vi "AlGaInPAs_prep_run_cont_v09.vi"(2 "Debug Mode":bool, 3 "Elapsed Time(s)":dbl, 4 "State":enum16{"Edit", "Start", "Run", "End", "Idle"}(ring), 5 "Argument List In":string[](array[string])) -> (0 "Status Out":string, 1 "Argument List Out":string[](array[string]))   [LabVIEW 2011]
panel:
  out "Prep-In var":bool
  out "Prep-Ga var":bool
  out "Prep-Al var":bool
  out "Prep-P var":bool
  out "Prep-As var":bool
  out "prep_done":bool
  out "run started":bool
  out "first":bool=TRUE
  out "total time":dbl
  out "is OK?":bool
  out "AsH3?":bool
  out "PH3?":bool
  out "In?":bool
  out "Ga?":bool
  out "Al?":bool
  in  "Prep As":bool caption="Pre-run"
  in  "Prep P":bool caption="Pre-run"
  in  "Prep In":bool caption="Pre-run"
  in  "Prep Ga":bool caption="Pre-run"
  in  "prep_time":dbl caption="pre-run time (s)"
  in  "Prep Al":bool caption="Pre-run"
  in  "Run As":bool caption="Run"
  in  "AsH3 Flow":dbl caption="AsH3 Flow (0-10 sccm)" format="%.2f"
  in  "P Flow":dbl caption="P Flow (0-100 sccm)" format="%.2f"
  in  "Run P":bool caption="Run"
  in  "In Flow":dbl caption="In Flow (0-100 sscm)" format="%.2f"
  in  "Run In":bool caption="Run"
  in  "Run Ga":bool caption="Run"
  in  "Ga Flow":dbl caption="Ga Flow (0-10 sscm)" format="%.2f"
  in  "Run Al":bool caption="Run"
  in  "Al Flow":dbl caption="Al Flow (0-100 sscm)" format="%.2f"
  in  "Cancel":bool
  in  "OK":bool
  out "tTotal(s) 2":dbl
  # "Add pre-run time to run time in editor."
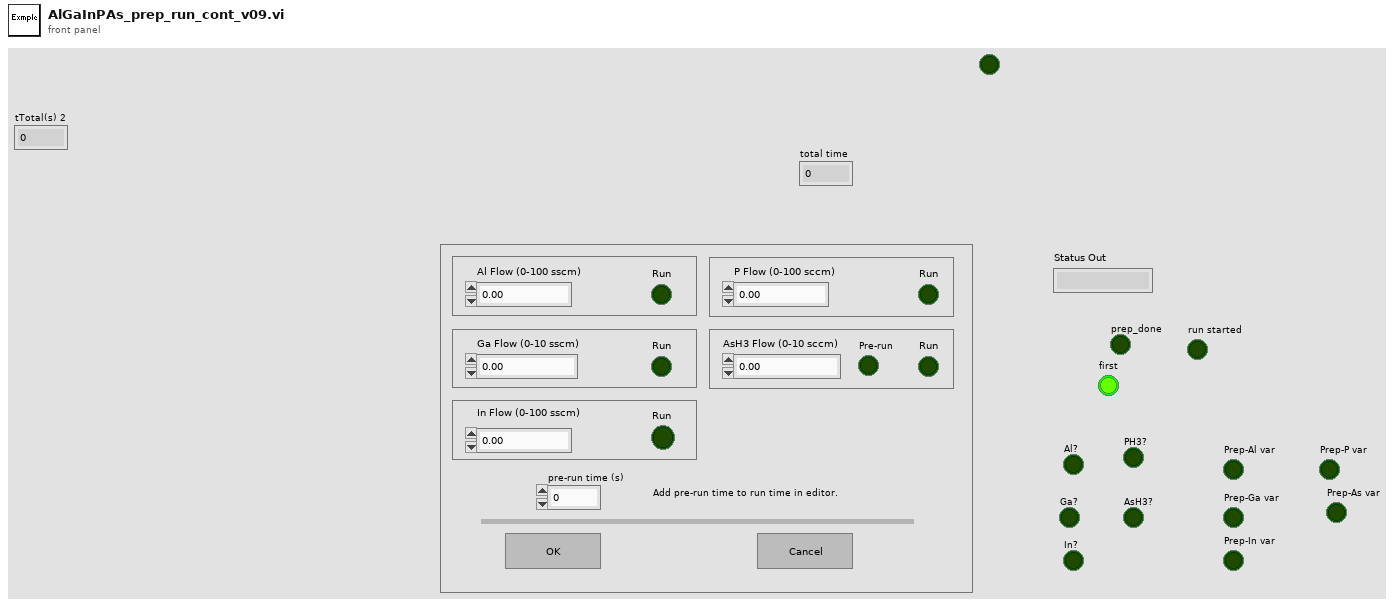
[diagram p1: front panel]
types:
  T1 = enum16{"Discrete", "Continuous", "Instantaneous", "Finite"}
  T2 = enum32{"Invalid", "Default", "Floating", "Floating/Auto-Hide", "Modal"}
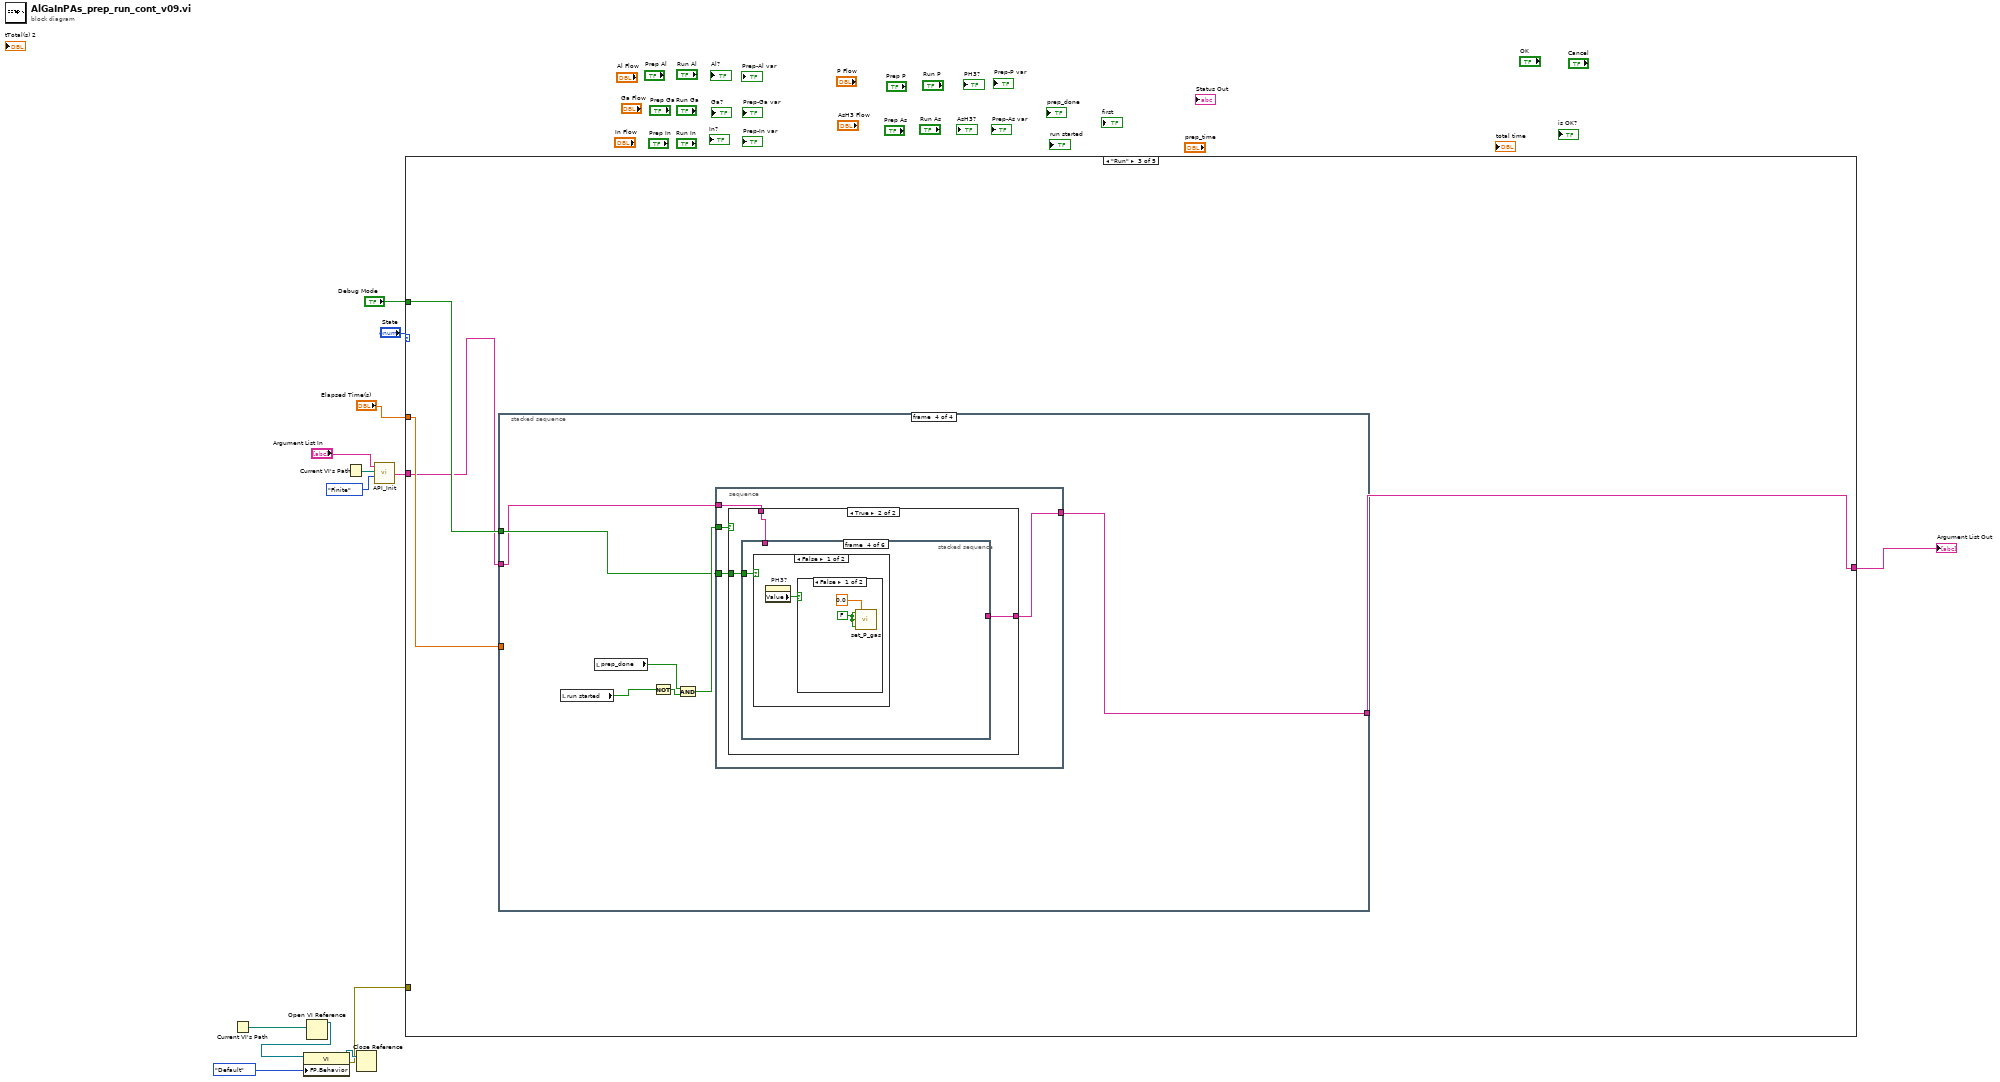
[diagram p0: block diagram]
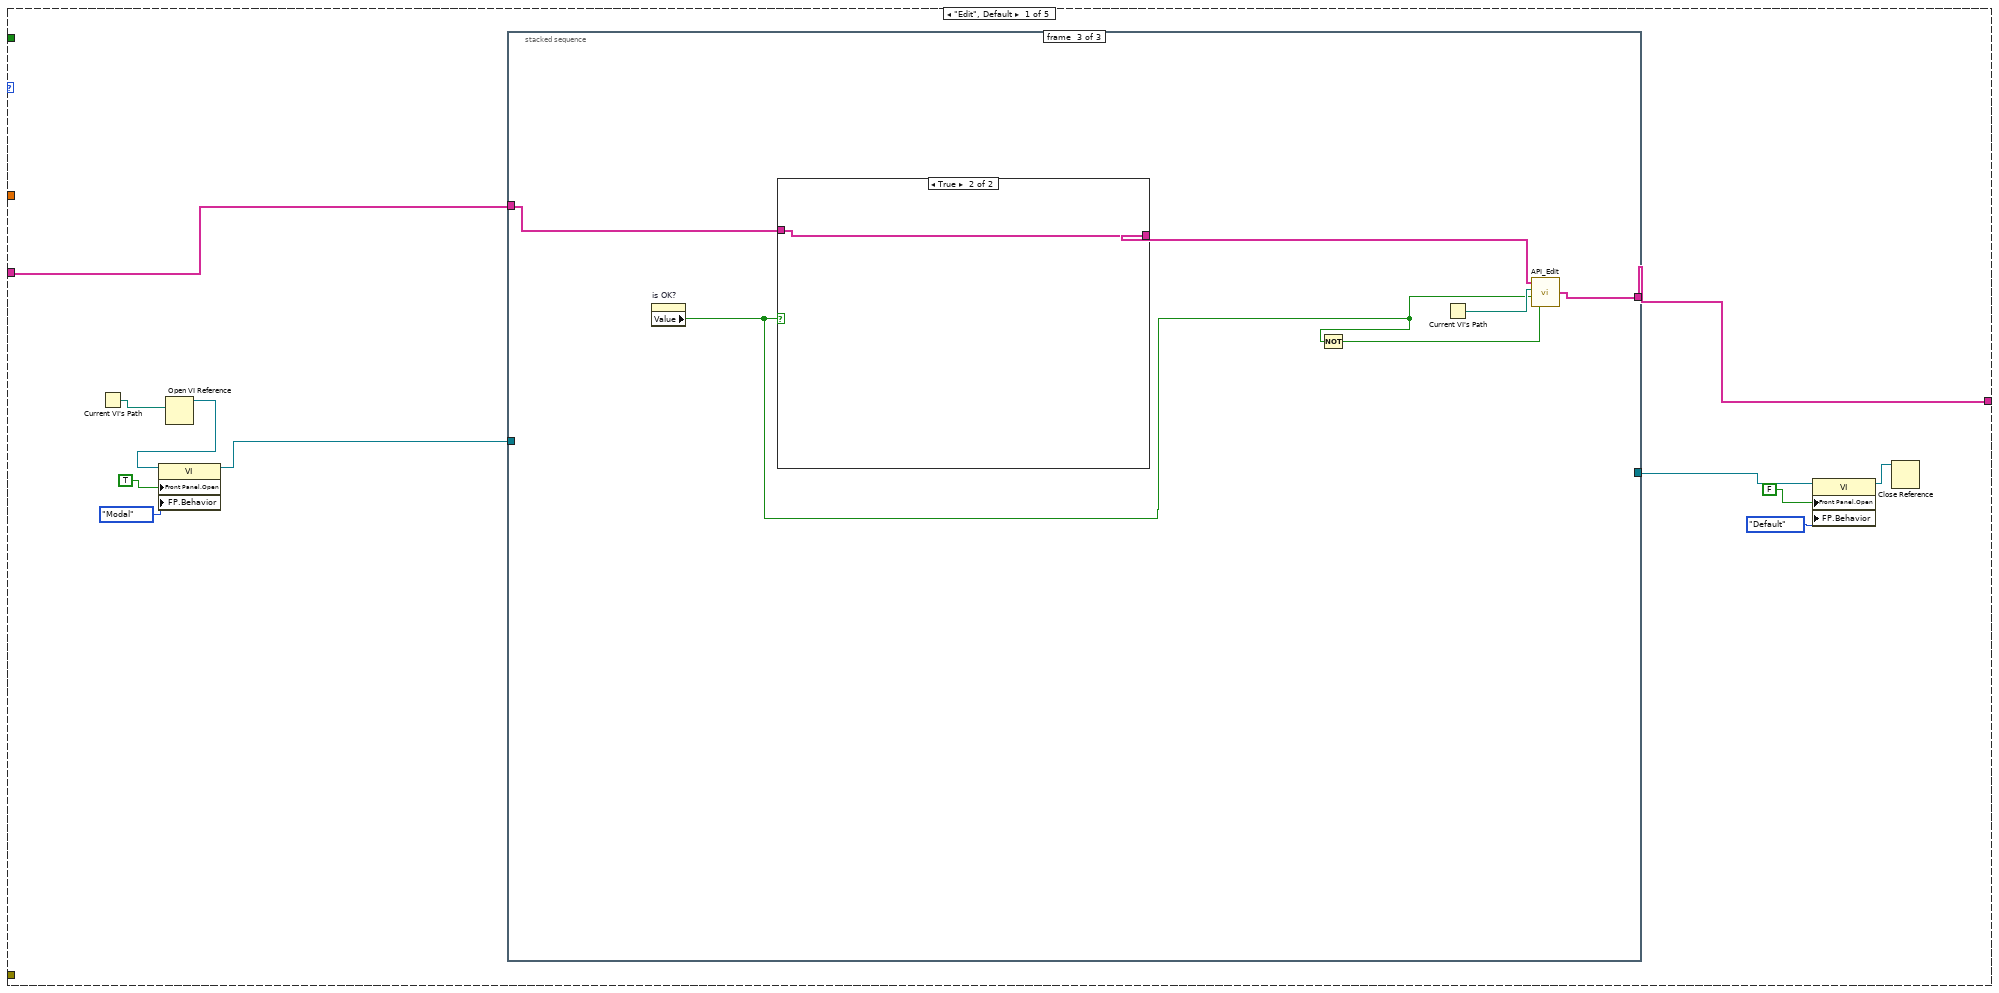
[diagram p2: hidden frame]
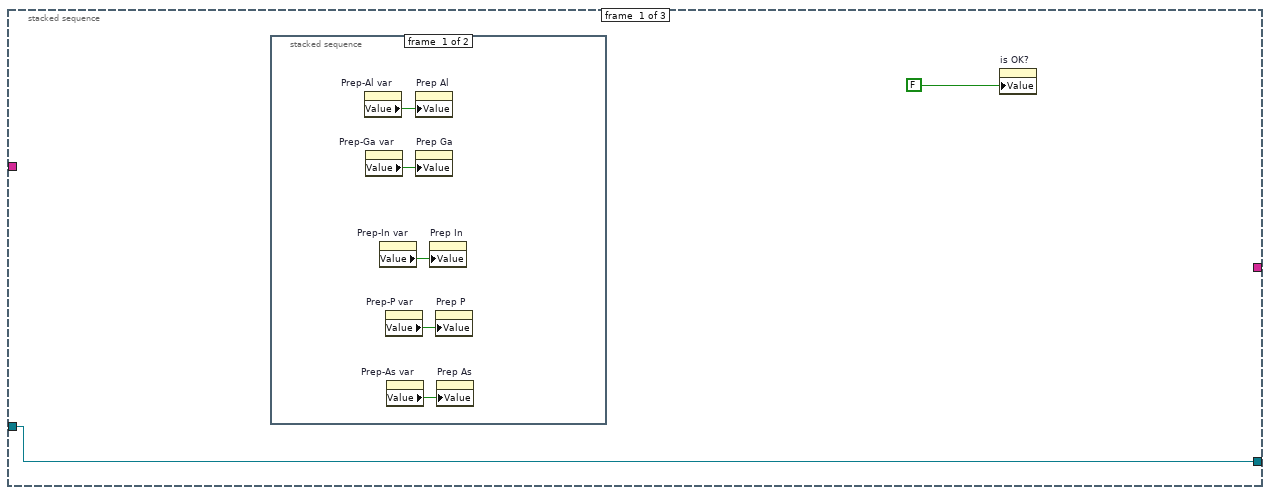
[diagram p3: hidden frame]
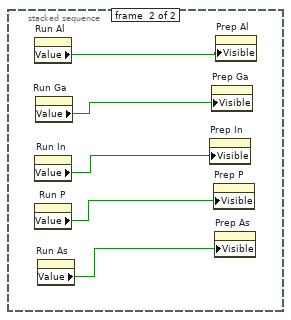
[diagram p4: hidden frame]
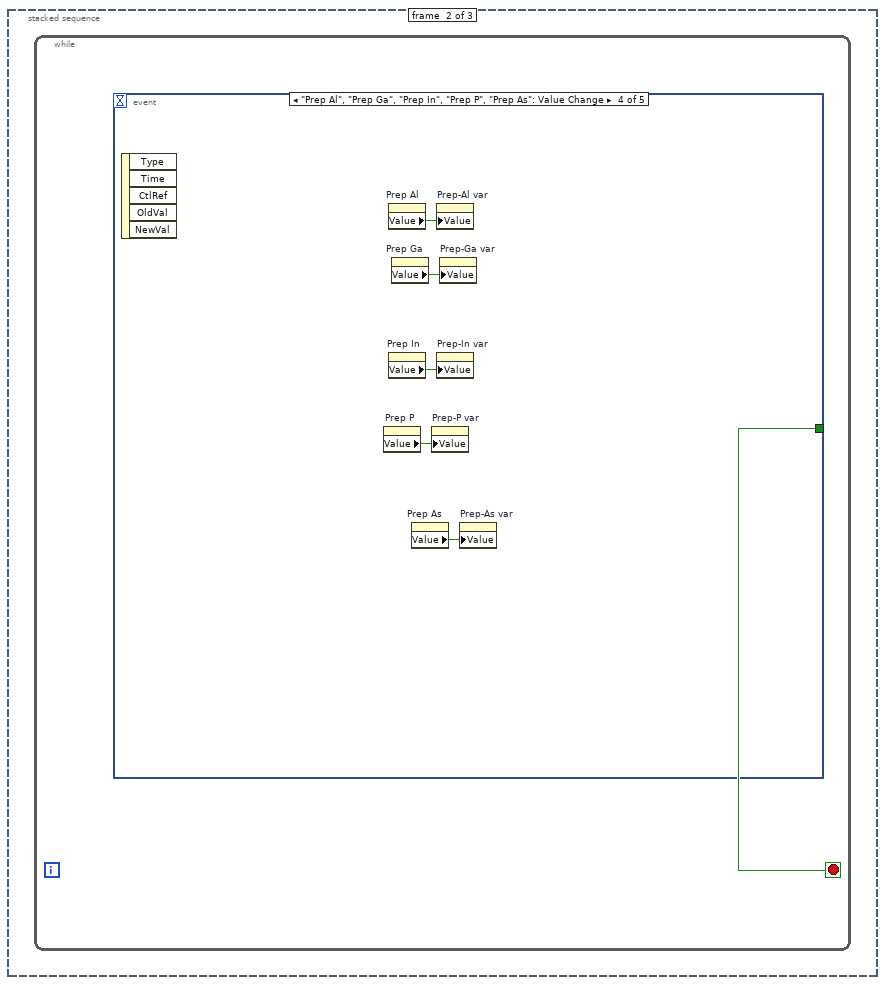
[diagram p5: hidden frame]
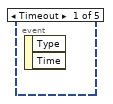
[diagram p6: hidden frame]
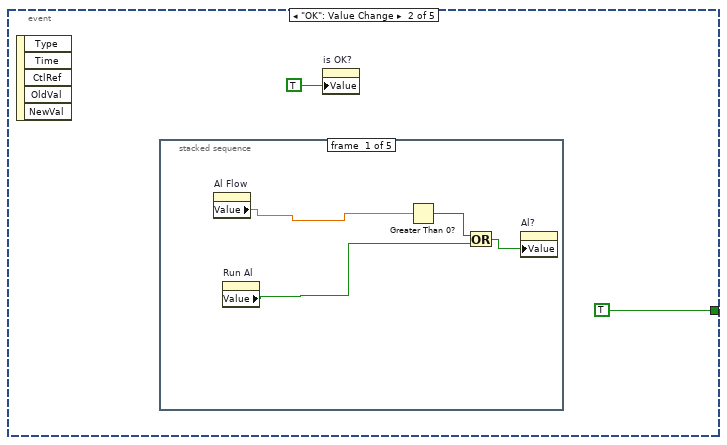
[diagram p7: hidden frame]
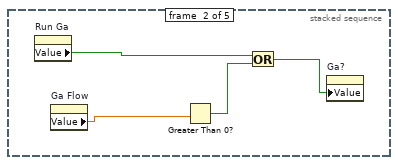
[diagram p8: hidden frame]
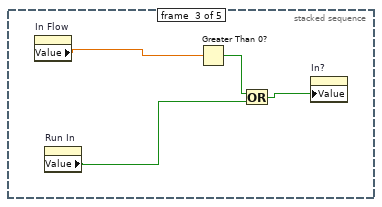
[diagram p9: hidden frame]
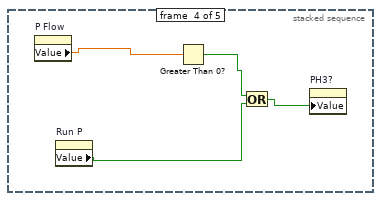
[diagram p10: hidden frame]
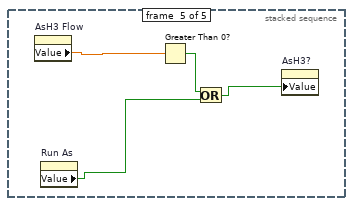
[diagram p11: hidden frame]
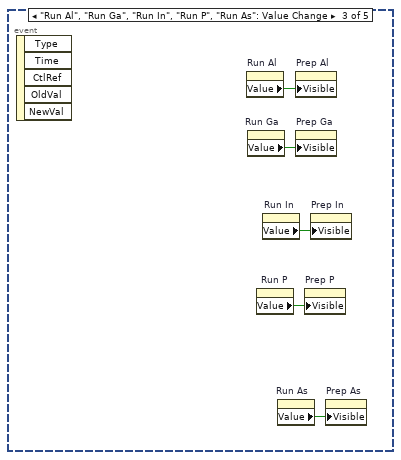
[diagram p12: hidden frame]
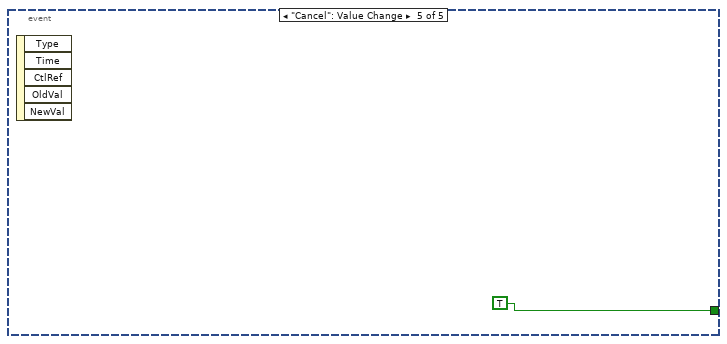
[diagram p13: hidden frame]
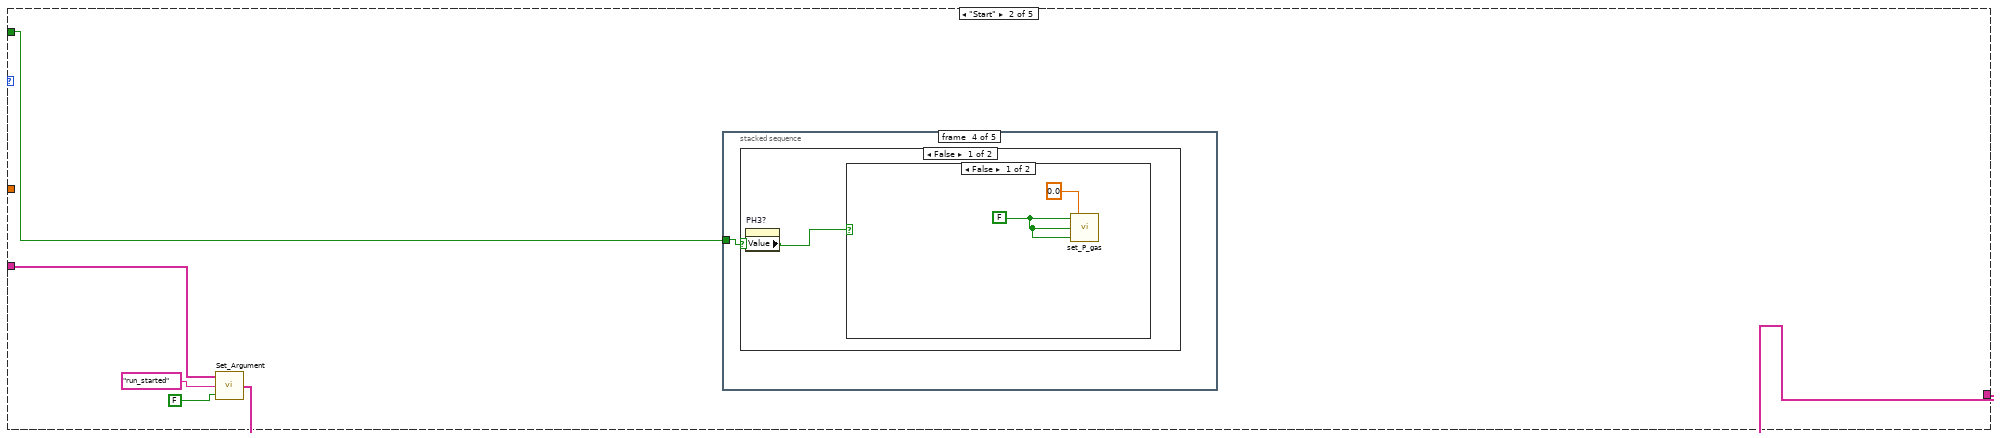
[diagram p15: hidden frame]
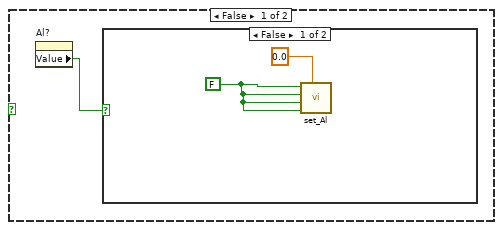
[diagram p17: hidden frame]
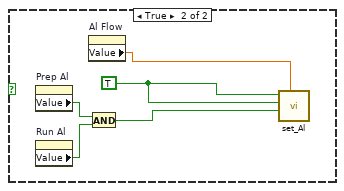
[diagram p18: hidden frame]
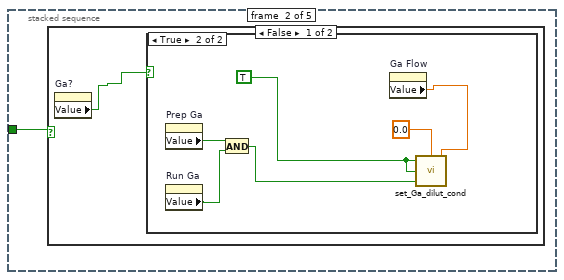
[diagram p19: hidden frame]
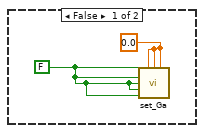
[diagram p20: hidden frame]
diagram:
  n1 = Current VI's Path() -> (path=w9:path)
  n2 = Open VI Reference(vi path=w9) -> (vi reference=w8:refnum<vi>)  [unwired: 1 in, 5 out]
  n3 = property class="VI"(reference=w8, "FP.Behavior"=T2."Default" ("Front Panel Window:Behavior")) -> (reference out=w6:refnum<vi>, error out=w5:errorcluster)  [unwired: 1 in]
  n4 = Current VI's Path() -> (path=w4:path)
  n5 = Close Reference(reference=w6) -> ()  [unwired: 1 in, 1 out]
  n6 = call "API_Init.vi"("API Mode"=T1."Finite", "VI Path"=w4, "Argument List In"="Argument List In") -> ("Argument List Out"=w1:string[])  [unwired: 1 in]
  n7 = case shown="\"Run\"" "State" {
    tunnel: "Debug Mode" -> [_ w79 w131 _ _]
    tunnel: "Elapsed Time(s)" -> [_ _ w133 _ _]
    tunnel: w1 -> [w15 w81 w130 w246 w247]
    tunnel: [w14 w80 w132 w246 w247] -> w10
    tunnel: w5 -> [_ _ _ _ _]
    frame "Edit", Default {
      n8 = Current VI's Path() -> (path=w20:path)
      n9 = Open VI Reference(vi path=w20) -> (vi reference=w19:refnum<vi>)  [unwired: 1 in, 5 out]
      n10 = property class="VI"(reference=w19, "Front Panel.Open"=TRUE ("Front Panel Window:Open"), "FP.Behavior"=T2."Modal" ("Front Panel Window:Behavior")) -> (reference out=w18:refnum<vi>)  [unwired: 1 in, 1 out]
      n11 = stacked-sequence {
        tunnel: w15 -> [_ _ w74]
        tunnel: w18 -> [w26 _ _]
        tunnel: [w26 _ _] -> w22
        tunnel: [_ _ w72] -> w14
        frame #0 {
          n12 = stacked-sequence {
            frame #0 {
              n13 = property on="Prep-Al var" class="Bool (strict)"() -> ("Value"=w31:bool)  [unwired: 2 in, 2 out]
              n14 = property on="Prep-Ga var" class="Bool (strict)"() -> ("Value"=w30:bool)  [unwired: 2 in, 2 out]
              n15 = property on="Prep-In var" class="Bool (strict)"() -> ("Value"=w29:bool)  [unwired: 2 in, 2 out]
              n16 = property on="Prep-P var" class="Bool (strict)"() -> ("Value"=w28:bool)  [unwired: 2 in, 2 out]
              n17 = property on="Prep-As var" class="Bool (strict)"() -> ("Value"=w27:bool)  [unwired: 2 in, 2 out]
              n18 = property on="Prep Al" class="Bool (strict)"("Value"=w31) -> ()  [unwired: 2 in, 2 out]
              n19 = property on="Prep Ga" class="Bool (strict)"("Value"=w30) -> ()  [unwired: 2 in, 2 out]
              n20 = property on="Prep In" class="Bool (strict)"("Value"=w29) -> ()  [unwired: 2 in, 2 out]
              n21 = property on="Prep P" class="Bool (strict)"("Value"=w28) -> ()  [unwired: 2 in, 2 out]
              n22 = property on="Prep As" class="Bool (strict)"("Value"=w27) -> ()  [unwired: 2 in, 2 out]
            }
            frame #1 {
              n23 = property on="Run Al" class="Bool (strict)"() -> ("Value"=w36:bool)  [unwired: 2 in, 2 out]
              n24 = property on="Run In" class="Bool (strict)"() -> ("Value"=w34:bool)  [unwired: 2 in, 2 out]
              n25 = property on="Run P" class="Bool (strict)"() -> ("Value"=w33:bool)  [unwired: 2 in, 2 out]
              n26 = property on="Run Ga" class="Bool (strict)"() -> ("Value"=w35:bool)  [unwired: 2 in, 2 out]
              n27 = property on="Run As" class="Bool (strict)"() -> ("Value"=w32:bool)  [unwired: 2 in, 2 out]
              n28 = property on="Prep In" class="Bool (strict)"("Visible"=w34) -> ()  [unwired: 2 in, 2 out]
              n29 = property on="Prep Ga" class="Bool (strict)"("Visible"=w35) -> ()  [unwired: 2 in, 2 out]
              n30 = property on="Prep P" class="Bool (strict)"("Visible"=w33) -> ()  [unwired: 2 in, 2 out]
              n31 = property on="Prep As" class="Bool (strict)"("Visible"=w32) -> ()  [unwired: 2 in, 2 out]
              n32 = property on="Prep Al" class="Bool (strict)"("Visible"=w36) -> ()  [unwired: 2 in, 2 out]
            }
          }
          n33 = property on="is OK?" class="Bool (strict)"("Value"=FALSE ("is OK?")) -> ()  [unwired: 2 in, 2 out]
        }
        frame #1 {
          n34 = while {
            stop <- w37 stop-if-true
            n35 = event shown="[3] \"Prep Al\", \"Prep Ga\", \"Prep In\", \"Prep P\", \"Prep As\": Value Change" {
              selector: _ -> [_ _ _ _ _]
              dyn-events: _ -> [_ _ _ _ _]
              timeout: _ -> [_ _ _ _ _]
              tunnel: [_ TRUE _ _ TRUE] -> w37
              event Timeout {
                n36 = event-data() -> ()  [unwired: 1 in, 2 out]
              }
              event "OK": Value Change {
                n37 = event-data() -> ()  [unwired: 1 in, 5 out]
                n38 = stacked-sequence {
                  frame #0 {
                    n39 = property on="Al Flow" class="DigNum (strict)"() -> ("Value"=w42:dbl)  [unwired: 2 in, 2 out]
                    n40 = property on="Run Al" class="Bool (strict)"() -> ("Value"=w41:bool)  [unwired: 2 in, 2 out]
                    n41 = Greater Than 0?(x=w42) -> (x > 0?=w43:bool)
                    n42 = Or(x=w43, y=w41) -> (x .or. y?=w40:bool)
                    n43 = property on="Al?" class="Bool (strict)"("Value"=w40) -> ()  [unwired: 2 in, 2 out]
                  }
                  frame #1 {
                    n44 = property on="Run Ga" class="Bool (strict)"() -> ("Value"=w45:bool)  [unwired: 2 in, 2 out]
                    n45 = property on="Ga Flow" class="DigNum (strict)"() -> ("Value"=w46:dbl)  [unwired: 2 in, 2 out]
                    n46 = Greater Than 0?(x=w46) -> (x > 0?=w47:bool)
                    n47 = Or(x=w45, y=w47) -> (x .or. y?=w44:bool)
                    n48 = property on="Ga?" class="Bool (strict)"("Value"=w44) -> ()  [unwired: 2 in, 2 out]
                  }
                  frame #2 {
                    n49 = property on="In Flow" class="DigNum (strict)"() -> ("Value"=w49:dbl)  [unwired: 2 in, 2 out]
                    n50 = property on="Run In" class="Bool (strict)"() -> ("Value"=w50:bool)  [unwired: 2 in, 2 out]
                    n51 = Greater Than 0?(x=w49) -> (x > 0?=w51:bool)
                    n52 = Or(x=w51, y=w50) -> (x .or. y?=w48:bool)
                    n53 = property on="In?" class="Bool (strict)"("Value"=w48) -> ()  [unwired: 2 in, 2 out]
                  }
                  frame #3 {
                    n54 = property on="P Flow" class="DigNum (strict)"() -> ("Value"=w54:dbl)  [unwired: 2 in, 2 out]
                    n55 = property on="Run P" class="Bool (strict)"() -> ("Value"=w53:bool)  [unwired: 2 in, 2 out]
                    n56 = Greater Than 0?(x=w54) -> (x > 0?=w55:bool)
                    n57 = Or(x=w55, y=w53) -> (x .or. y?=w52:bool)
                    n58 = property on="PH3?" class="Bool (strict)"("Value"=w52) -> ()  [unwired: 2 in, 2 out]
                  }
                  frame #4 {
                    n59 = property on="AsH3 Flow" class="DigNum (strict)"() -> ("Value"=w58:dbl)  [unwired: 2 in, 2 out]
                    n60 = property on="Run As" class="Bool (strict)"() -> ("Value"=w57:bool)  [unwired: 2 in, 2 out]
                    n61 = Greater Than 0?(x=w58) -> (x > 0?=w59:bool)
                    n62 = Or(x=w59, y=w57) -> (x .or. y?=w56:bool)
                    n63 = property on="AsH3?" class="Bool (strict)"("Value"=w56) -> ()  [unwired: 2 in, 2 out]
                  }
                }
                n64 = property on="is OK?" class="Bool (strict)"("Value"=TRUE ("is OK?")) -> ()  [unwired: 2 in, 2 out]
              }
              event "Run Al", "Run Ga", "Run In", "Run P", "Run As": Value Change {
                n65 = event-data() -> ()  [unwired: 1 in, 5 out]
                n66 = property on="Run Al" class="Bool (strict)"() -> ("Value"=w64:bool)  [unwired: 2 in, 2 out]
                n67 = property on="Run Ga" class="Bool (strict)"() -> ("Value"=w63:bool)  [unwired: 2 in, 2 out]
                n68 = property on="Run P" class="Bool (strict)"() -> ("Value"=w60:bool)  [unwired: 2 in, 2 out]
                n69 = property on="Run In" class="Bool (strict)"() -> ("Value"=w62:bool)  [unwired: 2 in, 2 out]
                n70 = property on="Run As" class="Bool (strict)"() -> ("Value"=w61:bool)  [unwired: 2 in, 2 out]
                n71 = property on="Prep Al" class="Bool (strict)"("Visible"=w64) -> ()  [unwired: 2 in, 2 out]
                n72 = property on="Prep Ga" class="Bool (strict)"("Visible"=w63) -> ()  [unwired: 2 in, 2 out]
                n73 = property on="Prep P" class="Bool (strict)"("Visible"=w60) -> ()  [unwired: 2 in, 2 out]
                n74 = property on="Prep In" class="Bool (strict)"("Visible"=w62) -> ()  [unwired: 2 in, 2 out]
                n75 = property on="Prep As" class="Bool (strict)"("Visible"=w61) -> ()  [unwired: 2 in, 2 out]
              }
              event "Prep Al", "Prep Ga", "Prep In", "Prep P", "Prep As": Value Change {
                n76 = event-data() -> ()  [unwired: 1 in, 5 out]
                n77 = property on="Prep P" class="Bool (strict)"() -> ("Value"=w66:bool)  [unwired: 2 in, 2 out]
                n78 = property on="Prep Al" class="Bool (strict)"() -> ("Value"=w69:bool)  [unwired: 2 in, 2 out]
                n79 = property on="Prep In" class="Bool (strict)"() -> ("Value"=w67:bool)  [unwired: 2 in, 2 out]
                n80 = property on="Prep Ga" class="Bool (strict)"() -> ("Value"=w68:bool)  [unwired: 2 in, 2 out]
                n81 = property on="Prep As" class="Bool (strict)"() -> ("Value"=w65:bool)  [unwired: 2 in, 2 out]
                n82 = property on="Prep-P var" class="Bool (strict)"("Value"=w66) -> ()  [unwired: 2 in, 2 out]
                n83 = property on="Prep-Al var" class="Bool (strict)"("Value"=w69) -> ()  [unwired: 2 in, 2 out]
                n84 = property on="Prep-In var" class="Bool (strict)"("Value"=w67) -> ()  [unwired: 2 in, 2 out]
                n85 = property on="Prep-Ga var" class="Bool (strict)"("Value"=w68) -> ()  [unwired: 2 in, 2 out]
                n86 = property on="Prep-As var" class="Bool (strict)"("Value"=w65) -> ()  [unwired: 2 in, 2 out]
              }
              event "Cancel": Value Change {
                n87 = event-data() -> ()  [unwired: 1 in, 5 out]
              }
            }
          }
        }
        frame #2 {
          n88 = property on="is OK?" class="Bool (strict)"() -> ("Value"=w71:bool)  [unwired: 2 in, 2 out]
          n89 = case shown="True" w71 {
            tunnel: w74 -> [w77 w78]
            tunnel: [w77 w78] -> w73
            frame False {
            }
            frame True {
            }
          }
          n90 = Not(x=w71) -> (.not. x?=w76:bool)
          n91 = Current VI's Path() -> (path=w75:path)
          n92 = call "API_Edit.vi"("Cancel"=w76, "OK"=w71, "VI Path"=w75, "Argument List In"=w73) -> ("Argument List Out"=w72:string[])
        }
      }
      n93 = property class="VI"(reference=w22, "Front Panel.Open"=FALSE ("Front Panel Window:Open"), "FP.Behavior"=T2."Default" ("Front Panel Window:Behavior")) -> (reference out=w23:refnum<vi>)  [unwired: 1 in, 1 out]
      n94 = Close Reference(reference=w23) -> ()  [unwired: 1 in, 1 out]
    }
    frame "Start" {
      n95 = call "Set_Argument.vi"("Enable"=FALSE, "Argument"="run_started", "Argument List In"=w81) -> ("Argument List Out"=w80:string[])
      n96 = stacked-sequence {
        tunnel: w79 -> [w84 w93 w103 w112 w121]
        frame #0 {
          n97 = case shown="True" w84 {
            frame False {
              n98 = property on="Al?" class="Bool (strict)"() -> ("Value"=w85:bool)  [unwired: 2 in, 2 out]
              n99 = case shown="False" w85 {
                frame False {
                  w86 = FALSE ("Al Active")
                  n100 = call "set_Al.vi"("ALMFC1"=0.0 ("Aluminum Flow"), "Remote"=w86, "Run"=w86, "Bubbler In"=w86, "Active"=w86) -> ()  [unwired: 5 out]
                }
                frame True {
                  w92 = TRUE ("Al Active")
                  n101 = property on="Prep Al" class="Bool (strict)"() -> ("Value"=w90:bool)  [unwired: 2 in, 2 out]
                  n102 = property on="Run Al" class="Bool (strict)"() -> ("Value"=w89:bool)  [unwired: 2 in, 2 out]
                  n103 = property on="Al Flow" class="DigNum (strict)"() -> ("Value"=w91:dbl)  [unwired: 2 in, 2 out]
                  n104 = And(x=w90, y=w89) -> (x .and. y?=w88:bool)
                  n105 = call "set_Al.vi"("ALMFC1"=w91, "Run"=w88, "Bubbler In"=w92, "Active"=w92) -> ()  [unwired: 1 in, 5 out]
                }
              }
            }
            frame True {
            }
          }
        }
        frame #1 {
          n106 = case shown="False" w93 {
            frame False {
              n107 = property on="Ga?" class="Bool (strict)"() -> ("Value"=w94:bool)  [unwired: 2 in, 2 out]
              n108 = case shown="True" w94 {
                frame False {
                  w96 = FALSE ("Ga Active")
                  w95 = 0.0 ("Ga Flow 1")
                  n109 = call "set_Ga.vi"("Active"=w96, "GAMFC3"=w95, "GAMFC2"=w95, "GAMFC1"=w95, "Bubbler In"=w96, "H2 Dilute"=w96, "Run"=w96, "Remote"=w96) -> ()  [unwired: 8 out]
                }
                frame True {
                  w102 = TRUE ("Ga Active")
                  n110 = property on="Prep Ga" class="Bool (strict)"() -> ("Value"=w99:bool)  [unwired: 2 in, 2 out]
                  n111 = property on="Run Ga" class="Bool (strict)"() -> ("Value"=w98:bool)  [unwired: 2 in, 2 out]
                  n112 = And(x=w99, y=w98) -> (x .and. y?=w97:bool)
                  n113 = property on="Ga Flow" class="DigNum (strict)"() -> ("Value"=w100:dbl)  [unwired: 2 in, 2 out]
                  n114 = call "set_Ga_dilut_cond.vi"("Ga flow (0-10 sccm)"=w100, "fDilution"=0.0, "Run"=w97, "Bubbler In"=w102, "Active"=w102) -> ()
                }
              }
            }
            frame True {
            }
          }
        }
        frame #2 {
          n115 = case shown="False" w103 {
            frame False {
              n116 = property on="In?" class="Bool (strict)"() -> ("Value"=w104:bool)  [unwired: 2 in, 2 out]
              n117 = case shown="True" w104 {
                frame False {
                  w106 = FALSE ("In Remote")
                  n118 = call "set_In.vi"("INMFC1"=0.0 ("Indium Flow"), "Remote"=w106, "Run"=w106, "Bubbler In"=w106, "Active"=w106) -> ()  [unwired: 5 out]
                }
                frame True {
                  w111 = TRUE ("In Run")
                  n119 = property on="Run In" class="Bool (strict)"() -> ("Value"=w108:bool)  [unwired: 2 in, 2 out]
                  n120 = property on="Prep In" class="Bool (strict)"() -> ("Value"=w109:bool)  [unwired: 2 in, 2 out]
                  n121 = And(x=w109, y=w108) -> (x .and. y?=w107:bool)
                  n122 = property on="In Flow" class="DigNum (strict)"() -> ("Value"=w110:dbl)  [unwired: 2 in, 2 out]
                  n123 = call "set_In.vi"("INMFC1"=w110, "Run"=w107, "Bubbler In"=w111, "Active"=w111) -> ()  [unwired: 1 in, 5 out]
                }
              }
            }
            frame True {
            }
          }
        }
        frame #3 {
          n124 = case shown="False" w112 {
            frame False {
              n125 = property on="PH3?" class="Bool (strict)"() -> ("Value"=w113:bool)  [unwired: 2 in, 2 out]
              n126 = case shown="False" w113 {
                frame False {
                  w114 = FALSE ("P_Gas Active")
                  n127 = call "set_P_gas.vi"("Run"=w114, "Gas In"=w114, "Active"=w114, "P_Gas Remote"=w114, "H2 Flush"=w114, "P_Gas Flow"=0.0) -> ()
                }
                frame True {
                  w120 = TRUE ("P_Gas Active")
                  n128 = property on="P Flow" class="DigNum (strict)"() -> ("Value"=w119:dbl)  [unwired: 2 in, 2 out]
                  n129 = property on="Prep P" class="Bool (strict)"() -> ("Value"=w118:bool)  [unwired: 2 in, 2 out]
                  n130 = property on="Run P" class="Bool (strict)"() -> ("Value"=w117:bool)  [unwired: 2 in, 2 out]
                  n131 = And(x=w118, y=w117) -> (x .and. y?=w116:bool)
                  n132 = call "set_P_gas.vi"("Active"=w120, "P_Gas Remote"=w116, "H2 Flush"=w120, "P_Gas Flow"=w119) -> ()  [unwired: 2 in]
                }
              }
            }
            frame True {
            }
          }
        }
        frame #4 {
          n133 = case shown="False" w121 {
            frame False {
              n134 = property on="AsH3?" class="Bool (strict)"() -> ("Value"=w122:bool)  [unwired: 2 in, 2 out]
              n135 = case shown="True" w122 {
                frame False {
                  w123 = FALSE ("As_Gas Active")
                  n136 = call "set_As_gas.vi"("Active"=w123, "As_Gas Flow"=0.0, "Gas In"=w123, "H2 Flush"=w123, "Run"=w123, "Remote"=w123) -> ()  [unwired: 10 in]
                }
                frame True {
                  w129 = TRUE ("As_Gas Active")
                  n137 = property on="Prep As" class="Bool (strict)"() -> ("Value"=w126:bool)  [unwired: 2 in, 2 out]
                  n138 = property on="Run As" class="Bool (strict)"() -> ("Value"=w127:bool)  [unwired: 2 in, 2 out]
                  n139 = property on="AsH3 Flow" class="DigNum (strict)"() -> ("Value"=w128:dbl)  [unwired: 2 in, 2 out]
                  n140 = And(x=w126, y=w127) -> (x .and. y?=w125:bool)
                  n141 = call "set_As_gas.vi"("Active"=w129, "As_Gas Flow"=w128, "Gas In"=w129, "Run"=w125) -> ()  [unwired: 12 in]
                }
              }
            }
            frame True {
            }
          }
        }
      }
    }
    frame "Run" {
      n142 = stacked-sequence {
        tunnel: w133 -> [_ w138 _ _]
        tunnel: w130 -> [w135 _ _ w192]
        tunnel: [_ _ _ w191] -> w132
        tunnel: w131 -> [_ _ _ w193]
        frame #0 {
          n143 = call "Get_Argument.vi"("Argument"="run_started", "Argument List"=w135) -> ("Enabled"=w134:bool)
          n144 = local write "run started"(w134) -> ()
        }
        frame #1 {
          n145 = property on="prep_time" class="DigNum (strict)"() -> ("Value"=w139:dbl)  [unwired: 2 in, 2 out]
          n146 = Greater Or Equal?(x=w138, y=w139) -> (x >= y?=w137:bool)
          n147 = local write "prep_done"(w137) -> ()
        }
        frame #2 {
          n148 = local read "run started"() -> (w141:bool)
          n149 = Not(x=w141) -> (.not. x?=w140:bool)
          n150 = stacked-sequence {
            tunnel: w140 -> [w143 w147 w156 w165 w174 w183]
            frame #0 {
              n151 = case shown="True" w143 {
                tunnel: ["run: " "pre-run: "] -> w142
                frame False {
                }
                frame True {
                }
              }
              n152 = property on="Status Out" class="Str"("Value"=w142) -> ()  [unwired: 2 in, 2 out]
            }
            frame #1 {
              n153 = property on="Status Out" class="Str"() -> ("Value"=w153:string)  [unwired: 2 in, 2 out]
              n154 = property on="Al?" class="Bool (strict)"() -> ("Value"=w154:bool)  [unwired: 2 in, 2 out]
              n155 = property on="Run Al" class="Bool (strict)"() -> ("Value"=w146:bool)  [unwired: 2 in, 2 out]
              n156 = property on="Prep Al" class="Bool (strict)"() -> ("Value"=w148:bool)  [unwired: 2 in, 2 out]
              n157 = call "flow_strings.vi"("string in"=w153, "is first in?"=TRUE, "use source?"=w154, "name"="Al", "run source?"=w146, "prep source?"=w148, "is prep?"=w147) -> ("string out"=w152:string, "is first out?"=w151:bool)
              n158 = property on="Status Out" class="Str"("Value"=w152) -> ()  [unwired: 2 in, 2 out]
              n159 = property on="first" class="Bool (strict)"("Value"=w151) -> ()  [unwired: 2 in, 2 out]
            }
            frame #2 {
              n160 = property on="first" class="Bool (strict)"() -> ("Value"=w159:bool)  [unwired: 2 in, 2 out]
              n161 = property on="Status Out" class="Str"() -> ("Value"=w162:string)  [unwired: 2 in, 2 out]
              n162 = property on="Ga?" class="Bool (strict)"() -> ("Value"=w160:bool)  [unwired: 2 in, 2 out]
              n163 = property on="Run Ga" class="Bool (strict)"() -> ("Value"=w155:bool)  [unwired: 2 in, 2 out]
              n164 = property on="Prep Ga" class="Bool (strict)"() -> ("Value"=w157:bool)  [unwired: 2 in, 2 out]
              n165 = call "flow_strings.vi"("string in"=w162, "is first in?"=w159, "use source?"=w160, "name"="Ga", "run source?"=w155, "prep source?"=w157, "is prep?"=w156) -> ("string out"=w163:string, "is first out?"=w158:bool)
              n166 = property on="Status Out" class="Str"("Value"=w163) -> ()  [unwired: 2 in, 2 out]
              n167 = property on="first" class="Bool (strict)"("Value"=w158) -> ()  [unwired: 2 in, 2 out]
            }
            frame #3 {
              n168 = property on="first" class="Bool (strict)"() -> ("Value"=w169:bool)  [unwired: 2 in, 2 out]
              n169 = property on="Status Out" class="Str"() -> ("Value"=w171:string)  [unwired: 2 in, 2 out]
              n170 = property on="In?" class="Bool (strict)"() -> ("Value"=w172:bool)  [unwired: 2 in, 2 out]
              n171 = property on="Run In" class="Bool (strict)"() -> ("Value"=w164:bool)  [unwired: 2 in, 2 out]
              n172 = property on="Prep In" class="Bool (strict)"() -> ("Value"=w166:bool)  [unwired: 2 in, 2 out]
              n173 = call "flow_strings.vi"("string in"=w171, "is first in?"=w169, "use source?"=w172, "name"="In", "run source?"=w164, "prep source?"=w166, "is prep?"=w165) -> ("string out"=w168:string, "is first out?"=w167:bool)
              n174 = property on="Status Out" class="Str"("Value"=w168) -> ()  [unwired: 2 in, 2 out]
              n175 = property on="first" class="Bool (strict)"("Value"=w167) -> ()  [unwired: 2 in, 2 out]
            }
            frame #4 {
              n176 = property on="first" class="Bool (strict)"() -> ("Value"=w177:bool)  [unwired: 2 in, 2 out]
              n177 = property on="Status Out" class="Str"() -> ("Value"=w179:string)  [unwired: 2 in, 2 out]
              n178 = property on="PH3?" class="Bool (strict)"() -> ("Value"=w180:bool)  [unwired: 2 in, 2 out]
              n179 = property on="Run P" class="Bool (strict)"() -> ("Value"=w173:bool)  [unwired: 2 in, 2 out]
              n180 = property on="Prep P" class="Bool (strict)"() -> ("Value"=w175:bool)  [unwired: 2 in, 2 out]
              n181 = call "flow_strings.vi"("string in"=w179, "is first in?"=w177, "use source?"=w180, "name"="P", "run source?"=w173, "prep source?"=w175, "is prep?"=w174) -> ("string out"=w178:string, "is first out?"=w176:bool)
              n182 = property on="Status Out" class="Str"("Value"=w178) -> ()  [unwired: 2 in, 2 out]
              n183 = property on="first" class="Bool (strict)"("Value"=w176) -> ()  [unwired: 2 in, 2 out]
            }
            frame #5 {
              n184 = property on="first" class="Bool (strict)"() -> ("Value"=w186:bool)  [unwired: 2 in, 2 out]
              n185 = property on="Status Out" class="Str"() -> ("Value"=w188:string)  [unwired: 2 in, 2 out]
              n186 = property on="AsH3?" class="Bool (strict)"() -> ("Value"=w189:bool)  [unwired: 2 in, 2 out]
              n187 = property on="Run As" class="Bool (strict)"() -> ("Value"=w182:bool)  [unwired: 2 in, 2 out]
              n188 = property on="Prep As" class="Bool (strict)"() -> ("Value"=w184:bool)  [unwired: 2 in, 2 out]
              n189 = call "flow_strings.vi"("string in"=w188, "is first in?"=w186, "use source?"=w189, "name"="As", "run source?"=w182, "prep source?"=w184, "is prep?"=w183) -> ("string out"=w185:string, "is first out?"=w187:bool)
              n190 = property on="Status Out" class="Str"("Value"=w185) -> ()  [unwired: 2 in, 2 out]
              n191 = property on="first" class="Bool (strict)"("Value"=w187) -> ()  [unwired: 2 in, 2 out]
            }
          }
        }
        frame #3 {
          n192 = local read "run started"() -> (w196:bool)
          n193 = local read "prep_done"() -> (w194:bool)
          n194 = Not(x=w196) -> (.not. x?=w197:bool)
          n195 = And(x=w194, y=w197) -> (x .and. y?=w195:bool)
          n196 = stacked-sequence {
            tunnel: w195 -> [w201]
            tunnel: w193 -> [w200]
            tunnel: w192 -> [w199]
            tunnel: [w198] -> w191
            frame #0 {
              n197 = case shown="True" w201 {
                tunnel: w200 -> [_ w205]
                tunnel: w199 -> [w202 w204]
                tunnel: [w202 w203] -> w198
                frame False {
                }
                frame True {
                  n198 = stacked-sequence {
                    tunnel: w205 -> [w206 w213 w221 w228 w235 _]
                    tunnel: w204 -> [_ _ _ _ _ w243]
                    tunnel: [_ _ _ _ _ w242] -> w203
                    frame #0 {
                      n199 = case shown="False" w206 {
                        frame False {
                          n200 = property on="Al?" class="Bool (strict)"() -> ("Value"=w207:bool)  [unwired: 2 in, 2 out]
                          n201 = case shown="True" w207 {
                            frame False {
                              w208 = FALSE ("Al Active")
                              n202 = call "set_Al.vi"("ALMFC1"=0.0 ("Aluminum Flow"), "Remote"=w208, "Run"=w208, "Bubbler In"=w208, "Active"=w208) -> ()  [unwired: 5 out]
                            }
                            frame True {
                              w212 = TRUE ("Al Active")
                              n203 = property on="Al Flow" class="DigNum (strict)"() -> ("Value"=w211:dbl)  [unwired: 2 in, 2 out]
                              n204 = property on="Run Al" class="Bool (strict)"() -> ("Value"=w210:bool)  [unwired: 2 in, 2 out]
                              n205 = call "set_Al.vi"("ALMFC1"=w211, "Run"=w210, "Bubbler In"=w212, "Active"=w212) -> ()  [unwired: 1 in, 5 out]
                            }
                          }
                        }
                        frame True {
                        }
                      }
                    }
                    frame #1 {
                      n206 = case shown="False" w213 {
                        frame False {
                          n207 = property on="Ga?" class="Bool (strict)"() -> ("Value"=w214:bool)  [unwired: 2 in, 2 out]
                          n208 = case shown="False" w214 {
                            frame False {
                              w216 = FALSE ("Ga Active")
                              w215 = 0.0 ("Ga Flow 1")
                              n209 = call "set_Ga.vi"("Active"=w216, "GAMFC3"=w215, "GAMFC2"=w215, "GAMFC1"=w215, "Bubbler In"=w216, "H2 Dilute"=w216, "Run"=w216, "Remote"=w216) -> ()  [unwired: 8 out]
                            }
                            frame True {
                              w220 = TRUE ("Ga Active")
                              n210 = property on="Ga Flow" class="DigNum (strict)"() -> ("Value"=w217:dbl)  [unwired: 2 in, 2 out]
                              n211 = property on="Run Ga" class="Bool (strict)"() -> ("Value"=w218:bool)  [unwired: 2 in, 2 out]
                              n212 = call "set_Ga_dilut_cond.vi"("Ga flow (0-10 sccm)"=w217, "fDilution"=0.0, "Run"=w218, "Bubbler In"=w220, "Active"=w220) -> ()
                            }
                          }
                        }
                        frame True {
                        }
                      }
                    }
                    frame #2 {
                      n213 = case shown="False" w221 {
                        frame False {
                          n214 = property on="In?" class="Bool (strict)"() -> ("Value"=w222:bool)  [unwired: 2 in, 2 out]
                          n215 = case shown="True" w222 {
                            frame False {
                              w224 = FALSE ("In Remote")
                              n216 = call "set_In.vi"("INMFC1"=0.0 ("Indium Flow"), "Remote"=w224, "Run"=w224, "Bubbler In"=w224, "Active"=w224) -> ()  [unwired: 5 out]
                            }
                            frame True {
                              w227 = TRUE ("In Run")
                              n217 = property on="Run In" class="Bool (strict)"() -> ("Value"=w225:bool)  [unwired: 2 in, 2 out]
                              n218 = property on="In Flow" class="DigNum (strict)"() -> ("Value"=w226:dbl)  [unwired: 2 in, 2 out]
                              n219 = call "set_In.vi"("INMFC1"=w226, "Run"=w225, "Bubbler In"=w227, "Active"=w227) -> ()  [unwired: 1 in, 5 out]
                            }
                          }
                        }
                        frame True {
                        }
                      }
                    }
                    frame #3 {
                      n220 = case shown="False" w228 {
                        frame False {
                          n221 = property on="PH3?" class="Bool (strict)"() -> ("Value"=w229:bool)  [unwired: 2 in, 2 out]
                          n222 = case shown="False" w229 {
                            frame False {
                              w230 = FALSE ("P_Gas Active")
                              n223 = call "set_P_gas.vi"("Run"=w230, "Gas In"=w230, "Active"=w230, "P_Gas Remote"=w230, "H2 Flush"=w230, "P_Gas Flow"=0.0) -> ()
                            }
                            frame True {
                              w234 = TRUE ("P_Gas Active")
                              n224 = property on="P Flow" class="DigNum (strict)"() -> ("Value"=w233:dbl)  [unwired: 2 in, 2 out]
                              n225 = property on="Run P" class="Bool (strict)"() -> ("Value"=w232:bool)  [unwired: 2 in, 2 out]
                              n226 = call "set_P_gas.vi"("Active"=w234, "P_Gas Remote"=w232, "H2 Flush"=w234, "P_Gas Flow"=w233) -> ()  [unwired: 2 in]
                            }
                          }
                        }
                        frame True {
                        }
                      }
                    }
                    frame #4 {
                      n227 = case shown="False" w235 {
                        frame False {
                          n228 = property on="AsH3?" class="Bool (strict)"() -> ("Value"=w236:bool)  [unwired: 2 in, 2 out]
                          n229 = case shown="True" w236 {
                            frame False {
                              w237 = FALSE ("As_Gas Active")
                              n230 = call "set_As_gas.vi"("Active"=w237, "As_Gas Flow"=0.0, "Gas In"=w237, "H2 Flush"=w237, "Run"=w237, "Remote"=w237) -> ()  [unwired: 10 in]
                            }
                            frame True {
                              w240 = TRUE ("As_Gas Active")
                              n231 = property on="Run As" class="Bool (strict)"() -> ("Value"=w239:bool)  [unwired: 2 in, 2 out]
                              n232 = property on="AsH3 Flow" class="DigNum (strict)"() -> ("Value"=w241:dbl)  [unwired: 2 in, 2 out]
                              n233 = call "set_As_gas.vi"("Active"=w240, "As_Gas Flow"=w241, "Gas In"=w240, "Run"=w239) -> ()  [unwired: 12 in]
                            }
                          }
                        }
                        frame True {
                        }
                      }
                    }
                    frame #5 {
                      n234 = call "Set_Argument.vi"("Enable"=TRUE, "Argument"="run_started", "Argument List In"=w243) -> ("Argument List Out"=w242:string[])
                    }
                  }
                }
              }
            }
          }
        }
      }
    }
    frame "End" {
    }
    frame "Idle" {
    }
  }
  "Argument List Out" <- w10
